vi "StatusReq.vi"(1 "aDATA in":u8[](array[numeric])) -> ()   [LabVIEW 2017]
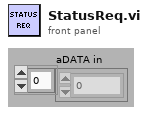
[diagram p1: front panel]
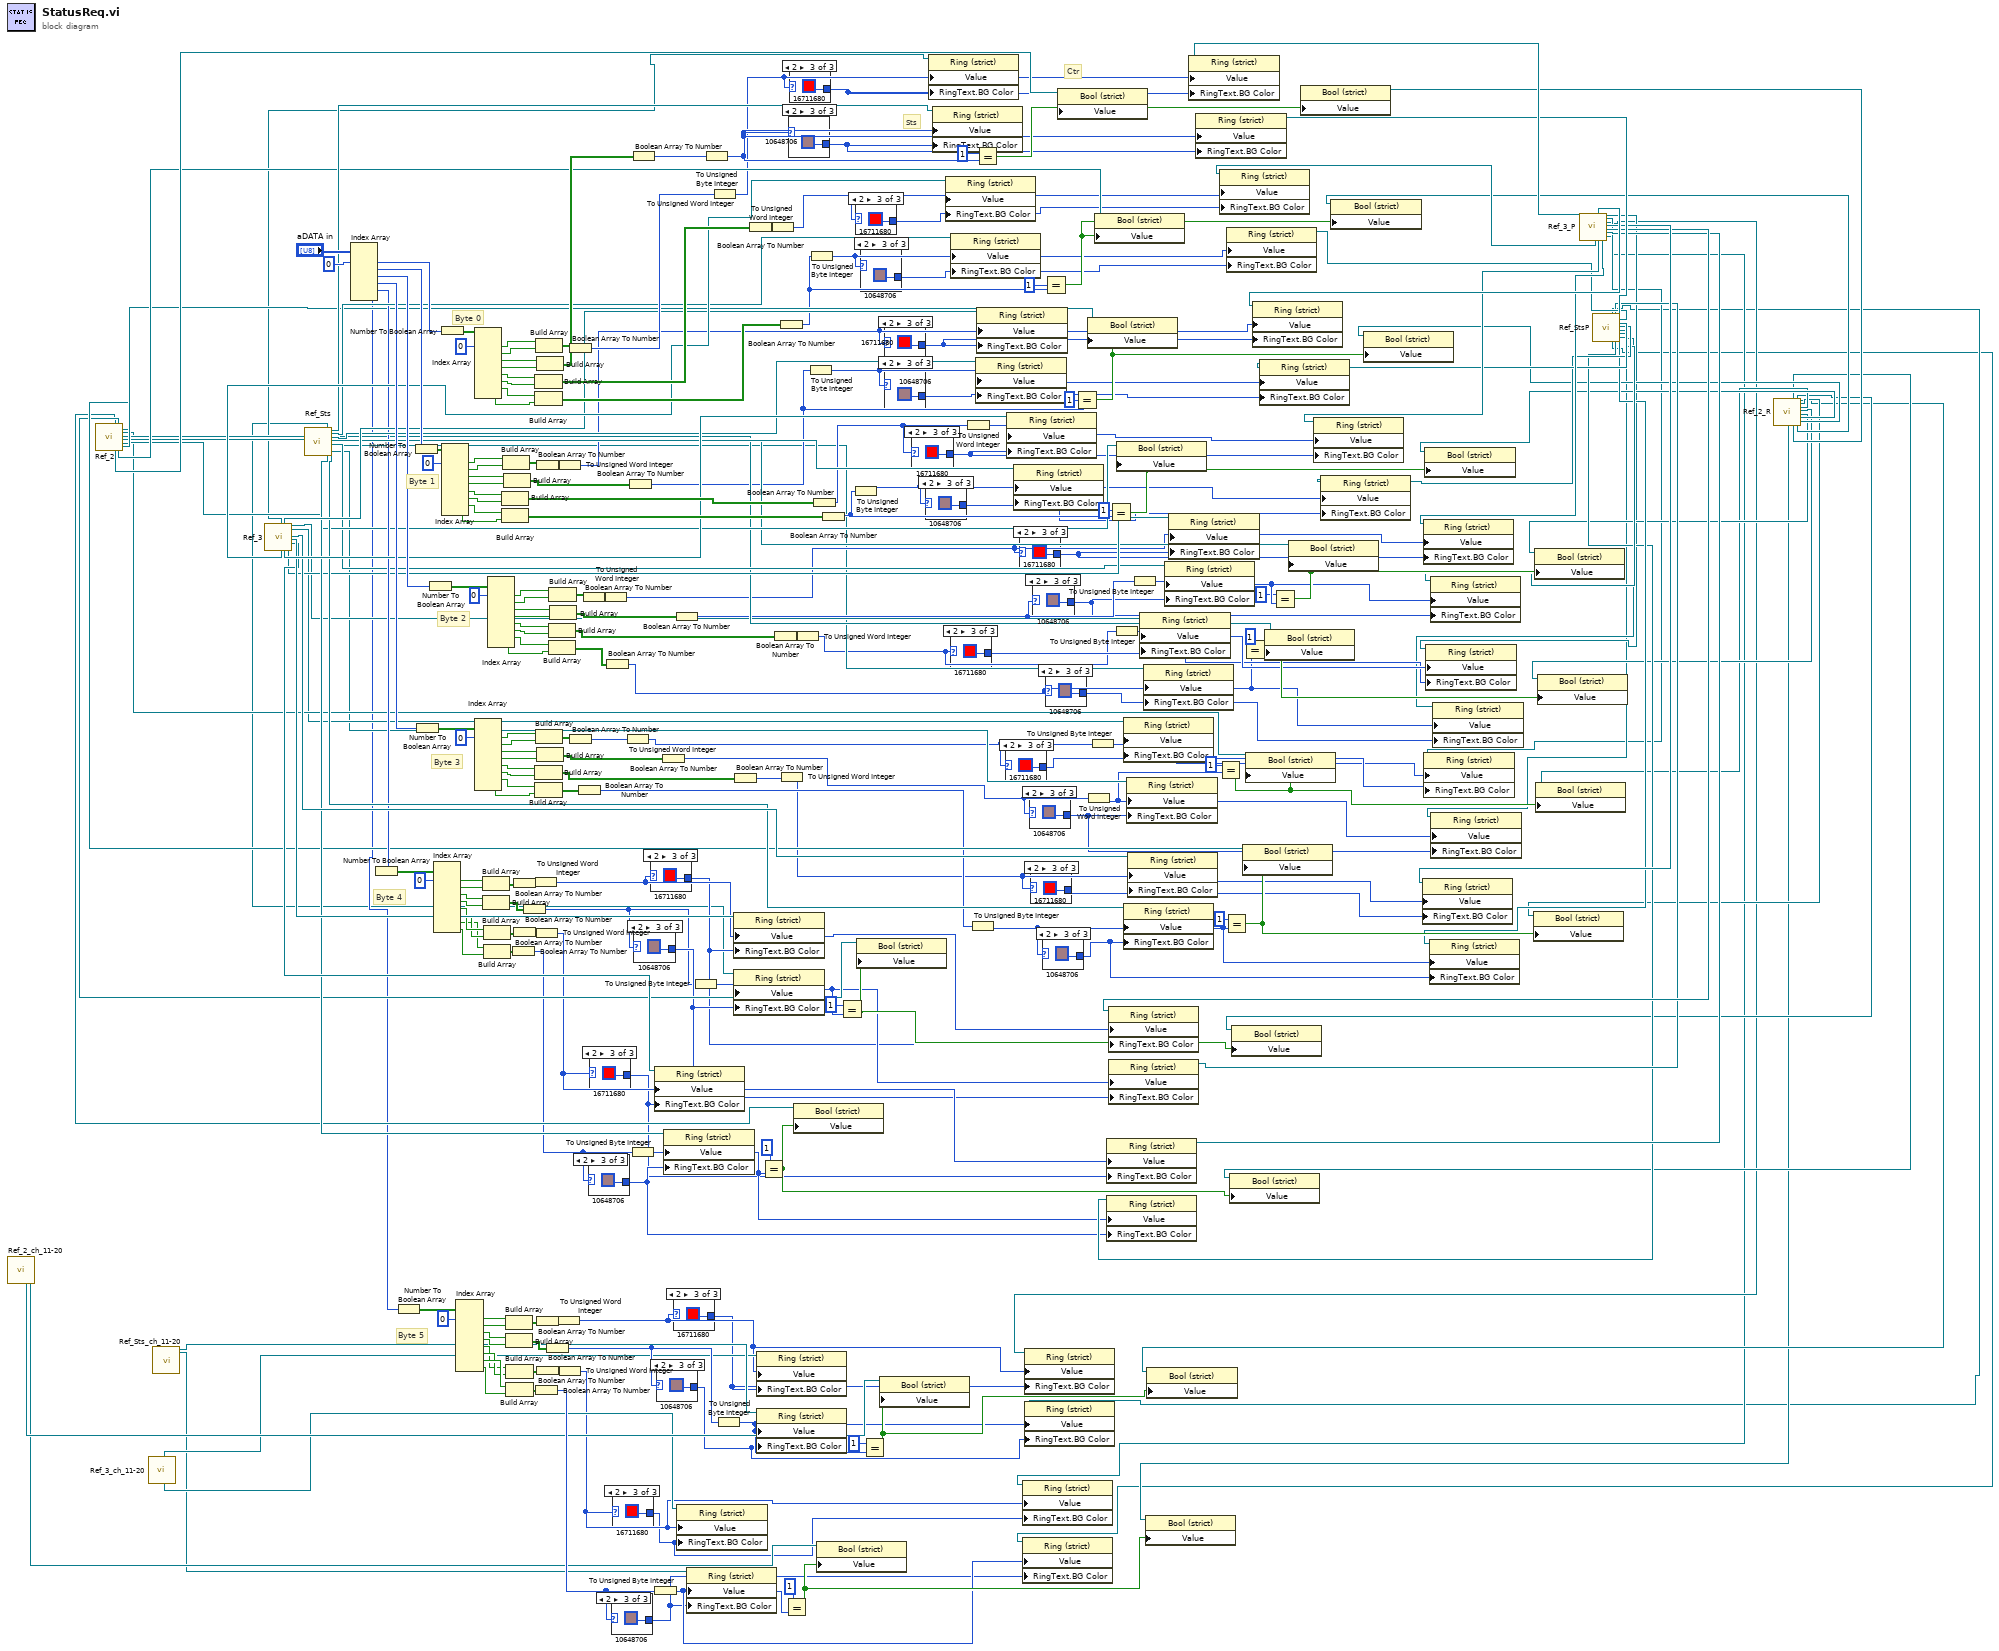
[diagram p0: block diagram]
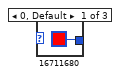
[diagram p2: hidden frame]
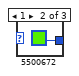
[diagram p3: hidden frame]
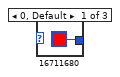
[diagram p4: hidden frame]
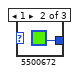
[diagram p5: hidden frame]
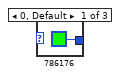
[diagram p6: hidden frame]
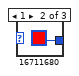
[diagram p7: hidden frame]
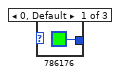
[diagram p8: hidden frame]
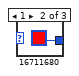
[diagram p9: hidden frame]
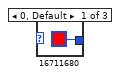
[diagram p10: hidden frame]
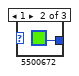
[diagram p11: hidden frame]
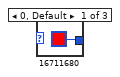
[diagram p12: hidden frame]
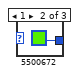
[diagram p13: hidden frame]
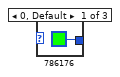
[diagram p14: hidden frame]
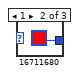
[diagram p15: hidden frame]
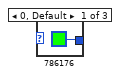
[diagram p16: hidden frame]
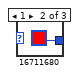
[diagram p17: hidden frame]
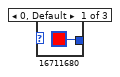
[diagram p18: hidden frame]
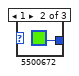
[diagram p19: hidden frame]
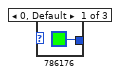
[diagram p20: hidden frame]
diagram:
  # "Trip ch12"
  # "Trip ch11"
  # "Byte 5"
  # "Trip ch10"
  # "Trip ch9"
  # "Trip ch8"
  # "trip ch7"
  # "trip ch6"
  # "Trip ch5"
  # "Trip ch4"
  # "Trip ch3"
  # "Trip ch2"
  # "Ctr"
  # "trip ch1"
  # "Sts"
  # "Byte 4"
  # "Byte 3"
  # "Byte 2"
  # "Byte 1"
  # "Byte 0"
  n1 = call "Ref_2_ch_11-20.vi"() -> ("Control  Ch 11 out"=w23:refnum<vi>, "Control  Ch 12 out"=w22:refnum<vi>)  [unwired: 17 in, 9 out]
  n2 = call "Ref_2.vi"() -> ("Control  Ch 10 out"=w158:refnum<vi>, "Control  Ch 1 out"=w164:refnum<vi>, "Control  Ch 9 out"=w159:refnum<vi>, "Control  Ch 2 out"=w163:refnum<vi>, "Control  Ch 8 out"=w160:refnum<vi>, "Control  Ch 7 out"=w86:refnum<vi>, "Control  Ch 6 out"=w154:refnum<vi>, "Control  Ch 5 out"=w155:refnum<vi>, "Control  Ch 4 out"=w161:refnum<vi>, "Control  Ch 3 out"=w162:refnum<vi>)  [unwired: 17 in, 1 out]
  n3 = call "Ref_3_ch_11-20.vi"() -> ("Trip  Ch 11 out"=w19:refnum<vi>, "Trip  Ch 12 out"=w18:refnum<vi>)  [unwired: 18 in, 8 out]
  n4 = call "Ref_Sts_ch_11-20.vi"() -> ("Status Ch 11 out"=w20:refnum<vi>, "Status Ch 12 out"=w17:refnum<vi>)  [unwired: 18 in, 8 out]
  n5 = call "Ref_3.vi"() -> ("Trip  Ch 1 out"=w60:refnum<vi>, "Trip  Ch 2 out"=w193:refnum<vi>, "Trip  Ch 3 out"=w192:refnum<vi>, "Trip  Ch 4 out"=w191:refnum<vi>, "Trip  Ch 5 out"=w157:refnum<vi>, "Trip  Ch 6 out"=w59:refnum<vi>, "Trip  Ch 7 out"=w57:refnum<vi>, "Trip  Ch 8 out"=w190:refnum<vi>, "Trip  Ch 9 out"=w174:refnum<vi>, "Trip  Ch 10 out"=w166:refnum<vi>)  [unwired: 18 in]
  n6 = call "Ref_Sts.vi"() -> ("Status Ch9 out"=w21:refnum<vi>, "Status Ch10 out"=w165:refnum<vi>, "Status Ch1 out"=w189:refnum<vi>, "Status Ch2 out"=w188:refnum<vi>, "Status Ch3 out"=w187:refnum<vi>, "Status Ch4 out"=w186:refnum<vi>, "Status Ch5 out"=w156:refnum<vi>, "Status Ch6 out"=w58:refnum<vi>, "Status Ch7 out"=w56:refnum<vi>, "Status Ch8 out"=w185:refnum<vi>)  [unwired: 18 in]
  n7 = Index Array(array="aDATA in", index #1=0 ("index")) -> (element #1=w259:u8, element #2=w229:u8, element #3=w228:u8, element #4=w227:u8, element #5=w182:u8, element #6=w24:u8)  [unwired: 5 in]
  n8 = Number To Boolean Array(number=w182) -> (Boolean array=w184:bool[])
  n9 = Number To Boolean Array(number=w24) -> (Boolean array=w25:bool[])
  n10 = Number To Boolean Array(number=w229) -> (Boolean array=w244:bool[])
  n11 = Number To Boolean Array(number=w227) -> (Boolean array=w230:bool[])
  n12 = Number To Boolean Array(number=w228) -> (Boolean array=w243:bool[])
  n13 = Index Array(array=w184, index #1=0 ("index")) -> (element #1=w180:bool, element #2=w181:bool, element #3=w179:bool, element #4=w178:bool, element #5=w170:bool, element #6=w169:bool, element #7=w168:bool, element #8=w167:bool)  [unwired: 7 in]
  n14 = Number To Boolean Array(number=w259) -> (Boolean array=w258:bool[])
  n15 = Index Array(array=w244, index #1=0 ("index")) -> (element #1=w218:bool, element #2=w217:bool, element #3=w216:bool, element #4=w215:bool, element #5=w214:bool, element #6=w213:bool, element #7=w212:bool, element #8=w211:bool)  [unwired: 7 in]
  n16 = Index Array(array=w25, index #1=0 ("index")) -> (element #1=w28:bool, element #2=w27:bool, element #3=w29:bool, element #4=w30:bool, element #5=w37:bool, element #6=w38:bool, element #7=w39:bool, element #8=w40:bool)  [unwired: 7 in]
  n17 = Index Array(array=w258, index #1=0 ("index")) -> (element #1=w226:bool, element #2=w225:bool, element #3=w224:bool, element #4=w223:bool, element #5=w222:bool, element #6=w221:bool, element #7=w220:bool, element #8=w219:bool)  [unwired: 7 in]
  n18 = Index Array(array=w230, index #1=0 ("index")) -> (element #1=w202:bool, element #2=w201:bool, element #3=w200:bool, element #4=w199:bool, element #5=w198:bool, element #6=w197:bool, element #7=w196:bool, element #8=w195:bool)  [unwired: 7 in]
  n19 = Build Array(w180, w181) -> (w176:bool[])
  n20 = Build Array(w179, w178) -> (w175:bool[])
  n21 = Build Array(w170, w169) -> (w172:bool[])
  n22 = Build Array(w168, w167) -> (w173:bool[])
  n23 = Index Array(array=w243, index #1=0 ("index")) -> (element #1=w210:bool, element #2=w209:bool, element #3=w208:bool, element #4=w207:bool, element #5=w206:bool, element #6=w205:bool, element #7=w204:bool, element #8=w203:bool)  [unwired: 7 in]
  n24 = Build Array(w214, w213) -> (w249:bool[])
  n25 = Build Array(w212, w211) -> (w248:bool[])
  n26 = Build Array(w218, w217) -> (w246:bool[])
  n27 = Build Array(w216, w215) -> (w250:bool[])
  n28 = Build Array(w28, w27) -> (w32:bool[])
  n29 = Build Array(w29, w30) -> (w33:bool[])
  n30 = Build Array(w37, w38) -> (w35:bool[])
  n31 = Build Array(w39, w40) -> (w34:bool[])
  n32 = Boolean Array To Number(Boolean array=w173) -> (number=w76:u32)
  n33 = Boolean Array To Number(Boolean array=w176) -> (number=w177:u32)
  n34 = Boolean Array To Number(Boolean array=w172) -> (number=w171:u32)
  n35 = Boolean Array To Number(Boolean array=w175) -> (number=w72:u32)
  n36 = To Unsigned Word Integer(number=w177) -> (unsigned 16bit integer=w79:u16)
  n37 = To Unsigned Word Integer(number=w171) -> (unsigned 16bit integer=w78:u16)
  n38 = Boolean Array To Number(Boolean array=w34) -> (number=w41:u32)
  n39 = Boolean Array To Number(Boolean array=w246) -> (number=w247:u32)
  n40 = Boolean Array To Number(Boolean array=w32) -> (number=w31:u32)
  n41 = Boolean Array To Number(Boolean array=w35) -> (number=w36:u32)
  n42 = Build Array(w222, w221) -> (w252:bool[])
  n43 = Build Array(w220, w219) -> (w253:bool[])
  n44 = Build Array(w198, w197) -> (w234:bool[])
  n45 = Build Array(w196, w195) -> (w194:bool[])
  n46 = Build Array(w226, w225) -> (w256:bool[])
  n47 = Build Array(w202, w201) -> (w232:bool[])
  n48 = Build Array(w224, w223) -> (w251:bool[])
  n49 = Build Array(w200, w199) -> (w235:bool[])
  n50 = Boolean Array To Number(Boolean array=w33) -> (number=w42:u32)
  n51 = Build Array(w206, w205) -> (w237:bool[])
  n52 = Build Array(w204, w203) -> (w238:bool[])
  n53 = Build Array(w210, w209) -> (w241:bool[])
  n54 = Build Array(w208, w207) -> (w236:bool[])
  n55 = To Unsigned Word Integer(number=w31) -> (unsigned 16bit integer=w16:u16)
  n56 = To Unsigned Word Integer(number=w247) -> (unsigned 16bit integer=w102:u16)
  n57 = To Unsigned Word Integer(number=w36) -> (unsigned 16bit integer=w11:u16)
  n58 = Boolean Array To Number(Boolean array=w256) -> (number=w255:u32)
  n59 = Boolean Array To Number(Boolean array=w232) -> (number=w53:u32)
  n60 = Boolean Array To Number(Boolean array=w194) -> (number=w149:u32)
  n61 = Boolean Array To Number(Boolean array=w241) -> (number=w240:u32)
  n62 = case shown="2" w76 {
    tunnel: [u32 16711680 ("Color 2") u32 5500672 ("Color 2") u32 10648706 ("Color 2")] -> w75
    frame 0, Default {
    }
    frame 1 {
    }
    frame 2 {
    }
  }
  n63 = case shown="2" w78 {
    tunnel: [u32 786176 ("Color 2") u32 16711680 ("Color 2") u32 16711680 ("Color 2")] -> w74
    frame 0, Default {
    }
    frame 1 {
    }
    frame 2 {
    }
  }
  n64 = To Unsigned Word Integer(number=w240) -> (unsigned 16bit integer=w94:u16)
  n65 = Boolean Array To Number(Boolean array=w238) -> (number=w50:u32)
  n66 = case shown="2" w41 {
    tunnel: [u32 16711680 ("Color 2") u32 5500672 ("Color 2") u32 10648706 ("Color 2")] -> w7
    frame 0, Default {
    }
    frame 1 {
    }
    frame 2 {
    }
  }
  n67 = case shown="2" w11 {
    tunnel: [u32 786176 ("Color 2") u32 16711680 ("Color 2") u32 16711680 ("Color 2")] -> w10
    frame 0, Default {
    }
    frame 1 {
    }
    frame 2 {
    }
  }
  n68 = To Unsigned Word Integer(number=w53) -> (unsigned 16bit integer=w52:u16)
  n69 = Boolean Array To Number(Boolean array=w250) -> (number=w152:u32)
  n70 = To Unsigned Byte Integer(number=w76) -> (unsigned 8bit integer=w77:u8)
  n71 = Boolean Array To Number(Boolean array=w251) -> (number=w153:u32)
  n72 = case shown="2" w72 {
    tunnel: [u32 16711680 ("Color 2") u32 5500672 ("Color 2") u32 10648706 ("Color 2")] -> w73
    frame 0, Default {
    }
    frame 1 {
    }
    frame 2 {
    }
  }
  n73 = case shown="2" w79 {
    tunnel: [u32 786176 ("Color 2") u32 16711680 ("Color 2") u32 16711680 ("Color 2")] -> w71
    frame 0, Default {
    }
    frame 1 {
    }
    frame 2 {
    }
  }
  n74 = To Unsigned Byte Integer(number=w41) -> (unsigned 8bit integer=w8:u8)
  n75 = property class="Ring (strict)"(reference=w166, "Value"=w78, "RingText.BG Color"=w74) -> ()  [unwired: 1 in, 2 out]
  n76 = case shown="2" w42 {
    tunnel: [u32 16711680 ("Color 2") u32 5500672 ("Color 2") u32 10648706 ("Color 2")] -> w12
    frame 0, Default {
    }
    frame 1 {
    }
    frame 2 {
    }
  }
  n77 = Boolean Array To Number(Boolean array=w235) -> (number=w54:u32)
  n78 = property class="Ring (strict)"(reference=w165, "Value"=w77, "RingText.BG Color"=w75) -> ()  [unwired: 1 in, 2 out]
  n79 = Boolean Array To Number(Boolean array=w236) -> (number=w93:u32)
  n80 = case shown="2" w16 {
    tunnel: [u32 786176 ("Color 2") u32 16711680 ("Color 2") u32 16711680 ("Color 2")] -> w15
    frame 0, Default {
    }
    frame 1 {
    }
    frame 2 {
    }
  }
  n81 = property class="Ring (strict)"(reference=w18, "Value"=w11, "RingText.BG Color"=w10) -> ()  [unwired: 1 in, 2 out]
  n82 = property class="Ring (strict)"(reference=w17, "Value"=w8, "RingText.BG Color"=w7) -> ()  [unwired: 1 in, 2 out]
  n83 = To Unsigned Byte Integer(number=w72) -> (unsigned 8bit integer=w80:u8)
  n84 = To Unsigned Byte Integer(number=w153) -> (unsigned 8bit integer=w111:u8)
  n85 = To Unsigned Word Integer(number=w255) -> (unsigned 16bit integer=w109:u16)
  n86 = To Unsigned Byte Integer(number=w42) -> (unsigned 8bit integer=w13:u8)
  n87 = Boolean Array To Number(Boolean array=w234) -> (number=w233:u32)
  n88 = property class="Ring (strict)"(reference=w174, "Value"=w79, "RingText.BG Color"=w71) -> ()  [unwired: 1 in, 2 out]
  n89 = property class="Ring (strict)"(reference=w21, "Value"=w80, "RingText.BG Color"=w73) -> ()  [unwired: 1 in, 2 out]
  n90 = Boolean Array To Number(Boolean array=w252) -> (number=w254:u32)
  n91 = property class="Ring (strict)"(reference=w19, "Value"=w16, "RingText.BG Color"=w15) -> ()  [unwired: 1 in, 2 out]
  n92 = property class="Ring (strict)"(reference=w20, "Value"=w13, "RingText.BG Color"=w12) -> ()  [unwired: 1 in, 2 out]
  n93 = Equal?(x=u8 1, y=w77) -> (x = y?=w130:bool)
  n94 = To Unsigned Word Integer(number=w254) -> (unsigned 16bit integer=w107:u16)
  n95 = Boolean Array To Number(Boolean array=w237) -> (number=w239:u32)
  n96 = Boolean Array To Number(Boolean array=w253) -> (number=w150:u32)
  n97 = To Unsigned Word Integer(number=w233) -> (unsigned 16bit integer=w83:u16)
  n98 = Equal?(x=u8 1, y=w8) -> (x = y?=w9:bool)
  n99 = case shown="2" w111 {
    tunnel: [u32 16711680 ("Color 2") u32 5500672 ("Color 2") u32 10648706 ("Color 2")] -> w110
    frame 0, Default {
    }
    frame 1 {
    }
    frame 2 {
    }
  }
  n100 = case shown="2" w109 {
    tunnel: [u32 786176 ("Color 2") u32 16711680 ("Color 2") u32 16711680 ("Color 2")] -> w108
    frame 0, Default {
    }
    frame 1 {
    }
    frame 2 {
    }
  }
  n101 = To Unsigned Word Integer(number=w239) -> (unsigned 16bit integer=w55:u16)
  n102 = property class="Bool (strict)"(reference=w158, "Value"=w130) -> ()  [unwired: 1 in, 2 out]
  n103 = To Unsigned Byte Integer(number=w152) -> (unsigned 8bit integer=w103:u8)
  n104 = To Unsigned Byte Integer(number=w150) -> (unsigned 8bit integer=w106:u8)
  n105 = Boolean Array To Number(Boolean array=w249) -> (number=w98:u32)
  n106 = property class="Bool (strict)"(reference=w22, "Value"=w9) -> ()  [unwired: 1 in, 2 out]
  n107 = Boolean Array To Number(Boolean array=w248) -> (number=w151:u32)
  n108 = Equal?(x=u8 1, y=w80) -> (x = y?=w131:bool)
  n109 = To Unsigned Byte Integer(number=w151) -> (unsigned 8bit integer=w99:u8)
  n110 = case shown="2" w107 {
    tunnel: [u32 786176 ("Color 2") u32 16711680 ("Color 2") u32 16711680 ("Color 2")] -> w104
    frame 0, Default {
    }
    frame 1 {
    }
    frame 2 {
    }
  }
  n111 = property class="Bool (strict)"(reference=w159, "Value"=w131) -> ()  [unwired: 1 in, 2 out]
  n112 = case shown="2" w106 {
    tunnel: [u32 16711680 ("Color 2") u32 5500672 ("Color 2") u32 10648706 ("Color 2")] -> w105
    frame 0, Default {
    }
    frame 1 {
    }
    frame 2 {
    }
  }
  n113 = Equal?(x=u8 1, y=w13) -> (x = y?=w14:bool)
  n114 = property class="Bool (strict)"(reference=w23, "Value"=w14) -> ()  [unwired: 1 in, 2 out]
  n115 = case shown="2" w102 {
    tunnel: [u32 786176 ("Color 2") u32 16711680 ("Color 2") u32 16711680 ("Color 2")] -> w100
    frame 0, Default {
    }
    frame 1 {
    }
    frame 2 {
    }
  }
  n116 = case shown="2" w103 {
    tunnel: [u32 16711680 ("Color 2") u32 5500672 ("Color 2") u32 10648706 ("Color 2")] -> w101
    frame 0, Default {
    }
    frame 1 {
    }
    frame 2 {
    }
  }
  n117 = case shown="2" w98 {
    tunnel: [u32 786176 ("Color 2") u32 16711680 ("Color 2") u32 16711680 ("Color 2")] -> w97
    frame 0, Default {
    }
    frame 1 {
    }
    frame 2 {
    }
  }
  n118 = case shown="2" w99 {
    tunnel: [u32 16711680 ("Color 2") u32 5500672 ("Color 2") u32 10648706 ("Color 2")] -> w96
    frame 0, Default {
    }
    frame 1 {
    }
    frame 2 {
    }
  }
  n119 = property class="Ring (strict)"(reference=w60, "Value"=w109, "RingText.BG Color"=w108) -> ()  [unwired: 1 in, 2 out]
  n120 = property class="Ring (strict)"(reference=w189, "Value"=w111, "RingText.BG Color"=w110) -> ()  [unwired: 1 in, 2 out]
  n121 = property class="Ring (strict)"(reference=w193, "Value"=w107, "RingText.BG Color"=w104) -> ()  [unwired: 1 in, 2 out]
  n122 = property class="Ring (strict)"(reference=w188, "Value"=w106, "RingText.BG Color"=w105) -> ()  [unwired: 1 in, 2 out]
  n123 = case shown="2" w55 {
    tunnel: [u32 786176 ("Color 2") u32 16711680 ("Color 2") u32 16711680 ("Color 2")] -> w89
    frame 0, Default {
    }
    frame 1 {
    }
    frame 2 {
    }
  }
  n124 = To Unsigned Word Integer(number=w98) -> (unsigned 16bit integer=w142:u16)
  n125 = To Unsigned Byte Integer(number=w149) -> (unsigned 8bit integer=w84:u8)
  n126 = Equal?(x=u8 1, y=w111) -> (x = y?=w145:bool)
  n127 = property class="Ring (strict)"(reference=w187, "Value"=w103, "RingText.BG Color"=w101) -> ()  [unwired: 1 in, 2 out]
  n128 = property class="Ring (strict)"(reference=w192, "Value"=w102, "RingText.BG Color"=w100) -> ()  [unwired: 1 in, 2 out]
  n129 = case shown="2" w52 {
    tunnel: [u32 786176 ("Color 2") u32 16711680 ("Color 2") u32 16711680 ("Color 2")] -> w87
    frame 0, Default {
    }
    frame 1 {
    }
    frame 2 {
    }
  }
  n130 = property class="Ring (strict)"(reference=w191, "Value"=w142, "RingText.BG Color"=w97) -> ()  [unwired: 1 in, 2 out]
  n131 = property class="Ring (strict)"(reference=w186, "Value"=w99, "RingText.BG Color"=w96) -> ()  [unwired: 1 in, 2 out]
  n132 = case shown="2" w94 {
    tunnel: [u32 786176 ("Color 2") u32 16711680 ("Color 2") u32 16711680 ("Color 2")] -> w92
    frame 0, Default {
    }
    frame 1 {
    }
    frame 2 {
    }
  }
  n133 = case shown="2" w54 {
    tunnel: [u32 16711680 ("Color 2") u32 5500672 ("Color 2") u32 10648706 ("Color 2")] -> w85
    frame 0, Default {
    }
    frame 1 {
    }
    frame 2 {
    }
  }
  n134 = case shown="2" w83 {
    tunnel: [u32 786176 ("Color 2") u32 16711680 ("Color 2") u32 16711680 ("Color 2")] -> w81
    frame 0, Default {
    }
    frame 1 {
    }
    frame 2 {
    }
  }
  n135 = case shown="2" w93 {
    tunnel: [u32 16711680 ("Color 2") u32 5500672 ("Color 2") u32 10648706 ("Color 2")] -> w91
    frame 0, Default {
    }
    frame 1 {
    }
    frame 2 {
    }
  }
  n136 = Equal?(x=u32 1, y=w150) -> (x = y?=w144:bool)
  n137 = case shown="2" w84 {
    tunnel: [u32 16711680 ("Color 2") u32 5500672 ("Color 2") u32 10648706 ("Color 2")] -> w82
    frame 0, Default {
    }
    frame 1 {
    }
    frame 2 {
    }
  }
  n138 = case shown="2" w50 {
    tunnel: [u32 16711680 ("Color 2") u32 5500672 ("Color 2") u32 10648706 ("Color 2")] -> w88
    frame 0, Default {
    }
    frame 1 {
    }
    frame 2 {
    }
  }
  n139 = property class="Bool (strict)"(reference=w164, "Value"=w145) -> ()  [unwired: 1 in, 2 out]
  n140 = Equal?(x=u32 1, y=w152) -> (x = y?=w143:bool)
  n141 = To Unsigned Word Integer(number=w54) -> (unsigned 16bit integer=w51:u16)
  n142 = property class="Bool (strict)"(reference=w162, "Value"=w143) -> ()  [unwired: 1 in, 2 out]
  n143 = To Unsigned Byte Integer(number=w52) -> (unsigned 8bit integer=w45:u8)
  n144 = property class="Bool (strict)"(reference=w163, "Value"=w144) -> ()  [unwired: 1 in, 2 out]
  n145 = Equal?(x=u32 1, y=w151) -> (x = y?=w141:bool)
  n146 = To Unsigned Byte Integer(number=w55) -> (unsigned 8bit integer=w90:u8)
  n147 = property class="Bool (strict)"(reference=w161, "Value"=w141) -> ()  [unwired: 1 in, 2 out]
  n148 = property class="Ring (strict)"(reference=w57, "Value"=w45, "RingText.BG Color"=w87) -> ()  [unwired: 1 in, 2 out]
  n149 = property class="Ring (strict)"(reference=w185, "Value"=w84, "RingText.BG Color"=w82) -> ()  [unwired: 1 in, 2 out]
  n150 = property class="Ring (strict)"(reference=w56, "Value"=w51, "RingText.BG Color"=w85) -> ()  [unwired: 1 in, 2 out]
  n151 = property class="Ring (strict)"(reference=w190, "Value"=w83, "RingText.BG Color"=w81) -> ()  [unwired: 1 in, 2 out]
  n152 = To Unsigned Byte Integer(number=w93) -> (unsigned 8bit integer=w95:u8)
  n153 = property class="Ring (strict)"(reference=w59, "Value"=w90, "RingText.BG Color"=w89) -> ()  [unwired: 1 in, 2 out]
  n154 = property class="Ring (strict)"(reference=w58, "Value"=w50, "RingText.BG Color"=w88) -> ()  [unwired: 1 in, 2 out]
  n155 = property class="Ring (strict)"(reference=w156, "Value"=w95, "RingText.BG Color"=w91) -> ()  [unwired: 1 in, 2 out]
  n156 = property class="Ring (strict)"(reference=w157, "Value"=w94, "RingText.BG Color"=w92) -> ()  [unwired: 1 in, 2 out]
  n157 = Equal?(x=u8 1, y=w51) -> (x = y?=w138:bool)
  n158 = Equal?(x=u8 1, y=w84) -> (x = y?=w137:bool)
  n159 = Equal?(x=u8 1, y=w50) -> (x = y?=w139:bool)
  n160 = property class="Bool (strict)"(reference=w160, "Value"=w137) -> ()  [unwired: 1 in, 2 out]
  n161 = property class="Bool (strict)"(reference=w86, "Value"=w138) -> ()  [unwired: 1 in, 2 out]
  n162 = property class="Bool (strict)"(reference=w154, "Value"=w139) -> ()  [unwired: 1 in, 2 out]
  n163 = Equal?(x=u8 1, y=w95) -> (x = y?=w140:bool)
  n164 = property class="Bool (strict)"(reference=w155, "Value"=w140) -> ()  [unwired: 1 in, 2 out]
  n165 = call "Ref_3_P.vi"() -> ("Trip  Ch 1 out"=w148:refnum<vi>, "Trip  Ch 2 out"=w136:refnum<vi>, "Trip  Ch 3 out"=w135:refnum<vi>, "Trip  Ch 4 out"=w134:refnum<vi>, "Trip  Ch 5 out"=w133:refnum<vi>, "Trip  Ch 6 out"=w49:refnum<vi>, "Trip  Ch 7 out"=w46:refnum<vi>, "Trip  Ch 11 out"=w4:refnum<vi>, "Trip  Ch 8 out"=w132:refnum<vi>, "Trip  Ch 9 out"=w129:refnum<vi>, "Trip  Ch 10 out"=w128:refnum<vi>, "Trip  Ch 12 out"=w3:refnum<vi>)  [unwired: 16 in]
  n166 = property class="Ring (strict)"(reference=w3, "Value"=w11, "RingText.BG Color"=w10) -> ()  [unwired: 1 in, 2 out]
  n167 = property class="Ring (strict)"(reference=w4, "Value"=w16, "RingText.BG Color"=w15) -> ()  [unwired: 1 in, 2 out]
  n168 = property class="Ring (strict)"(reference=w128, "Value"=w78, "RingText.BG Color"=w74) -> ()  [unwired: 1 in, 2 out]
  n169 = property class="Ring (strict)"(reference=w129, "Value"=w79, "RingText.BG Color"=w71) -> ()  [unwired: 1 in, 2 out]
  n170 = property class="Ring (strict)"(reference=w148, "Value"=w109, "RingText.BG Color"=w108) -> ()  [unwired: 1 in, 2 out]
  n171 = property class="Ring (strict)"(reference=w136, "Value"=w107, "RingText.BG Color"=w104) -> ()  [unwired: 1 in, 2 out]
  n172 = property class="Ring (strict)"(reference=w135, "Value"=w102, "RingText.BG Color"=w100) -> ()  [unwired: 1 in, 2 out]
  n173 = property class="Ring (strict)"(reference=w134, "Value"=w142, "RingText.BG Color"=w97) -> ()  [unwired: 1 in, 2 out]
  n174 = property class="Ring (strict)"(reference=w132, "Value"=w83, "RingText.BG Color"=w81) -> ()  [unwired: 1 in, 2 out]
  n175 = property class="Ring (strict)"(reference=w133, "Value"=w94, "RingText.BG Color"=w92) -> ()  [unwired: 1 in, 2 out]
  n176 = property class="Ring (strict)"(reference=w46, "Value"=w45, "RingText.BG Color"=w87) -> ()  [unwired: 1 in, 2 out]
  n177 = property class="Ring (strict)"(reference=w49, "Value"=w90, "RingText.BG Color"=w89) -> ()  [unwired: 1 in, 2 out]
  n178 = call "Ref_StsP.vi"() -> ("Status Ch11 out"=w2:refnum<vi>, "Status Ch12 out"=w1:refnum<vi>, "Status Ch9 out"=w122:refnum<vi>, "Status Ch10 out"=w121:refnum<vi>, "Status Ch1 out"=w146:refnum<vi>, "Status Ch2 out"=w127:refnum<vi>, "Status Ch3 out"=w126:refnum<vi>, "Status Ch4 out"=w125:refnum<vi>, "Status Ch5 out"=w124:refnum<vi>, "Status Ch6 out"=w48:refnum<vi>, "Status Ch7 out"=w47:refnum<vi>, "Status Ch8 out"=w123:refnum<vi>)  [unwired: 16 in]
  n179 = property class="Ring (strict)"(reference=w1, "Value"=w8, "RingText.BG Color"=w7) -> ()  [unwired: 1 in, 2 out]
  n180 = property class="Ring (strict)"(reference=w2, "Value"=w13, "RingText.BG Color"=w12) -> ()  [unwired: 1 in, 2 out]
  n181 = property class="Ring (strict)"(reference=w121, "Value"=w77, "RingText.BG Color"=w75) -> ()  [unwired: 1 in, 2 out]
  n182 = property class="Ring (strict)"(reference=w122, "Value"=w80, "RingText.BG Color"=w73) -> ()  [unwired: 1 in, 2 out]
  n183 = property class="Ring (strict)"(reference=w146, "Value"=w111, "RingText.BG Color"=w110) -> ()  [unwired: 1 in, 2 out]
  n184 = property class="Ring (strict)"(reference=w127, "Value"=w106, "RingText.BG Color"=w105) -> ()  [unwired: 1 in, 2 out]
  n185 = property class="Ring (strict)"(reference=w126, "Value"=w103, "RingText.BG Color"=w101) -> ()  [unwired: 1 in, 2 out]
  n186 = property class="Ring (strict)"(reference=w125, "Value"=w99, "RingText.BG Color"=w96) -> ()  [unwired: 1 in, 2 out]
  n187 = property class="Ring (strict)"(reference=w123, "Value"=w84, "RingText.BG Color"=w82) -> ()  [unwired: 1 in, 2 out]
  n188 = property class="Ring (strict)"(reference=w124, "Value"=w95, "RingText.BG Color"=w91) -> ()  [unwired: 1 in, 2 out]
  n189 = property class="Ring (strict)"(reference=w47, "Value"=w51, "RingText.BG Color"=w85) -> ()  [unwired: 1 in, 2 out]
  n190 = property class="Ring (strict)"(reference=w48, "Value"=w50, "RingText.BG Color"=w88) -> ()  [unwired: 1 in, 2 out]
  n191 = call "Ref_2_R.vi"() -> ("Control  Ch 12 out"=w5:refnum<vi>, "Control  Ch 10 out"=w112:refnum<vi>, "Control  Ch 1 out"=w147:refnum<vi>, "Control  Ch 9 out"=w113:refnum<vi>, "Control  Ch 2 out"=w120:refnum<vi>, "Control  Ch 11 out"=w6:refnum<vi>, "Control  Ch 8 out"=w114:refnum<vi>, "Control  Ch 7 out"=w115:refnum<vi>, "Control  Ch 6 out"=w116:refnum<vi>, "Control  Ch 5 out"=w117:refnum<vi>, "Control  Ch 4 out"=w118:refnum<vi>, "Control  Ch 3 out"=w119:refnum<vi>)  [unwired: 15 in, 1 out]
  n192 = property class="Bool (strict)"(reference=w5, "Value"=w9) -> ()  [unwired: 1 in, 2 out]
  n193 = property class="Bool (strict)"(reference=w6, "Value"=w14) -> ()  [unwired: 1 in, 2 out]
  n194 = property class="Bool (strict)"(reference=w112, "Value"=w130) -> ()  [unwired: 1 in, 2 out]
  n195 = property class="Bool (strict)"(reference=w113, "Value"=w131) -> ()  [unwired: 1 in, 2 out]
  n196 = property class="Bool (strict)"(reference=w147, "Value"=w145) -> ()  [unwired: 1 in, 2 out]
  n197 = property class="Bool (strict)"(reference=w120, "Value"=w144) -> ()  [unwired: 1 in, 2 out]
  n198 = property class="Bool (strict)"(reference=w119, "Value"=w143) -> ()  [unwired: 1 in, 2 out]
  n199 = property class="Bool (strict)"(reference=w118, "Value"=w141) -> ()  [unwired: 1 in, 2 out]
  n200 = property class="Bool (strict)"(reference=w114, "Value"=w137) -> ()  [unwired: 1 in, 2 out]
  n201 = property class="Bool (strict)"(reference=w117, "Value"=w140) -> ()  [unwired: 1 in, 2 out]
  n202 = property class="Bool (strict)"(reference=w115, "Value"=w138) -> ()  [unwired: 1 in, 2 out]
  n203 = property class="Bool (strict)"(reference=w116, "Value"=w139) -> ()  [unwired: 1 in, 2 out]
